vi "XY Dialog - Update Selected Paths.vi"(7 "Data":variant, 8 "error in (no error)":errorcluster, 9 "Type":T1, 10 "Tree Browser Refnun":refnum<k24>, 11 "Dialog Data in":T2={"GraphData"={"Custom Data"=variant, "EventRegs"={"SystemChange"=refnum, "WorkspaceState"=refnum, "Graph"=refnum, "Wks&Dialog&Periodic"=refnum}, "References"={"X.Scale.Auto"=refnum, "Y.Scale.Auto"=refnum, "X.Scale.Once"=refnum, "Y.Scale.Once"=refnum, "LegendVis"=refnum, "Graph"=refnum}, "Persistent Data"={"Label"="", "Graph Props"={"Plots"=[], "Legend:Number of Rows"=0, "Scale Properties"={"X.Auto"=FALSE, "X.Min"=0.0, "X.Max"=0.0, "X.IgnoreTS"=FALSE, "X.Precision"=0, "X.Label:"="", "X.LabelVis"=FALSE, "X.DefLabel"=FALSE, "Y.Auto"=FALSE, "Y.Min"=0.0, "Y.Max"=0.0, "Y.Format"=0, "Y.Precision:"=0, "Y.Label:"="", "Y.LabelVis"=FALSE, "Y.DefLabel"=FALSE, "X.Format"=0}, "Legend:Visible"=TRUE, "BgColor"=0, "Last Plot Width"=0, "Resize"=FALSE}, "UDP Data"={"Decimation"=0, "UDP Buffer Size"=0, "History Length"=0.0, "Update Rate"=enum."15 Hz", "Channel Paths"=[], "Channel Names"=[]}}, "System"={"To Workspace"=refnum, "From Workspace"=refnum, "NIVS helper"=refnum, "Gtwy"="", "Root"=refnum, "Workspace"=refnum, "SystemStateRefs"={"CustDatRef"=refnum, "EvtRef"=refnum, "Target State User Event"=refnum}, "Connected?"=FALSE, "FromDialog"=refnum, "ErrFlag"=FALSE, "New"=FALSE, "ErrState"="", "Save"=FALSE, "Hold"=FALSE, "Periodic"=refnum, "ToDialog"=refnum, "DialogEventReg"=refnum, "UseSavedWidth"=FALSE, "TreeBrowserEventReg"=refnum, "UDPChannelStreamSession"=refnum, "Valid Channels?"=FALSE, "Update Graph"=refnum, "UDP Queue"=refnum, "Graph Update Queue"=refnum}, "GraphData"=[], "UDP Stream Active?"=FALSE}, "References"={"BgColor"=refnum, "Title"=refnum, "Waveforms"=refnum, "PointsPerPixel"=refnum, "Low"=refnum, "High"=refnum, "History"=refnum, "N"=refnum, "M"=refnum, "IgnTimeStamp"=refnum, "X.Precision"=refnum, "X.Label"=refnum, "X.Label.Default"=refnum, "X.Label.Visible"=refnum, "X.Autoscale"=refnum, "X.Max"=refnum, "X.Min"=refnum, "Y.Format"=refnum, "Y.Precision"=refnum, "Y.Label"=refnum, "Y.Label.Default"=refnum, "Y.Label.Visible"=refnum, "Y.Autoscale"=refnum, "Y.Max"=refnum, "Y.Min"=refnum, "rate"=refnum, "path"=refnum, "Alias TreeBrowser"=refnum, "Y Channel Listbox"=refnum, "X Channel Listbox"=refnum, "X.Format"=refnum, "X Next"=refnum, "Y Next"=refnum, "X Previous"=refnum, "Y Previous"=refnum, "Decimation"=refnum, "History Length"=refnum, "UDP Buffer Size"=refnum}, "Tree Selected Paths"=[], "SelectedIdx"=0, "dts"=[], "X Selected Paths"=[], "Y Selected Paths"=[]} {"GraphData"."Persistent Data"."Graph Props"."Scale Properties"."X.Format" items=["Decimal", "Scientific", "Engineering", "Binary", "Octal", "Hexadecimal", "Relative Time", "Time and Date", "SI", "Automatic"]; "GraphData"."Persistent Data"."Graph Props"."Scale Properties"."Y.Precision:" items=["0", "1", "2", "3", "4", "5", "6", "7"]; "GraphData"."Persistent Data"."Graph Props"."Scale Properties"."Y.Format" items=["Decimal", "Scientific", "Engineering", "Binary", "Octal", "Hexadecimal", "Relative Time", "Time and Date", "SI", "Automatic"]; "GraphData"."Persistent Data"."Graph Props"."Scale Properties"."X.Precision" items=["0", "1", "2", "3", "4", "5", "6", "7"]}) -> (0 "error out":errorcluster, 3 "Dialog Data out":T2={"GraphData"={"Custom Data"=variant, "EventRegs"={"SystemChange"=refnum, "WorkspaceState"=refnum, "Graph"=refnum, "Wks&Dialog&Periodic"=refnum}, "References"={"X.Scale.Auto"=refnum, "Y.Scale.Auto"=refnum, "X.Scale.Once"=refnum, "Y.Scale.Once"=refnum, "LegendVis"=refnum, "Graph"=refnum}, "Persistent Data"={"Label"="", "Graph Props"={"Plots"=[], "Legend:Number of Rows"=0, "Scale Properties"={"X.Auto"=FALSE, "X.Min"=0.0, "X.Max"=0.0, "X.IgnoreTS"=FALSE, "X.Precision"=0, "X.Label:"="", "X.LabelVis"=FALSE, "X.DefLabel"=FALSE, "Y.Auto"=FALSE, "Y.Min"=0.0, "Y.Max"=0.0, "Y.Format"=0, "Y.Precision:"=0, "Y.Label:"="", "Y.LabelVis"=FALSE, "Y.DefLabel"=FALSE, "X.Format"=0}, "Legend:Visible"=TRUE, "BgColor"=0, "Last Plot Width"=0, "Resize"=FALSE}, "UDP Data"={"Decimation"=0, "UDP Buffer Size"=0, "History Length"=0.0, "Update Rate"=enum."15 Hz", "Channel Paths"=[], "Channel Names"=[]}}, "System"={"To Workspace"=refnum, "From Workspace"=refnum, "NIVS helper"=refnum, "Gtwy"="", "Root"=refnum, "Workspace"=refnum, "SystemStateRefs"={"CustDatRef"=refnum, "EvtRef"=refnum, "Target State User Event"=refnum}, "Connected?"=FALSE, "FromDialog"=refnum, "ErrFlag"=FALSE, "New"=FALSE, "ErrState"="", "Save"=FALSE, "Hold"=FALSE, "Periodic"=refnum, "ToDialog"=refnum, "DialogEventReg"=refnum, "UseSavedWidth"=FALSE, "TreeBrowserEventReg"=refnum, "UDPChannelStreamSession"=refnum, "Valid Channels?"=FALSE, "Update Graph"=refnum, "UDP Queue"=refnum, "Graph Update Queue"=refnum}, "GraphData"=[], "UDP Stream Active?"=FALSE}, "References"={"BgColor"=refnum, "Title"=refnum, "Waveforms"=refnum, "PointsPerPixel"=refnum, "Low"=refnum, "High"=refnum, "History"=refnum, "N"=refnum, "M"=refnum, "IgnTimeStamp"=refnum, "X.Precision"=refnum, "X.Label"=refnum, "X.Label.Default"=refnum, "X.Label.Visible"=refnum, "X.Autoscale"=refnum, "X.Max"=refnum, "X.Min"=refnum, "Y.Format"=refnum, "Y.Precision"=refnum, "Y.Label"=refnum, "Y.Label.Default"=refnum, "Y.Label.Visible"=refnum, "Y.Autoscale"=refnum, "Y.Max"=refnum, "Y.Min"=refnum, "rate"=refnum, "path"=refnum, "Alias TreeBrowser"=refnum, "Y Channel Listbox"=refnum, "X Channel Listbox"=refnum, "X.Format"=refnum, "X Next"=refnum, "Y Next"=refnum, "X Previous"=refnum, "Y Previous"=refnum, "Decimation"=refnum, "History Length"=refnum, "UDP Buffer Size"=refnum}, "Tree Selected Paths"=[], "SelectedIdx"=0, "dts"=[], "X Selected Paths"=[], "Y Selected Paths"=[]} {"GraphData"."Persistent Data"."Graph Props"."Scale Properties"."X.Format" items=["Decimal", "Scientific", "Engineering", "Binary", "Octal", "Hexadecimal", "Relative Time", "Time and Date", "SI", "Automatic"]; "GraphData"."Persistent Data"."Graph Props"."Scale Properties"."Y.Precision:" items=["0", "1", "2", "3", "4", "5", "6", "7"]; "GraphData"."Persistent Data"."Graph Props"."Scale Properties"."Y.Format" items=["Decimal", "Scientific", "Engineering", "Binary", "Octal", "Hexadecimal", "Relative Time", "Time and Date", "SI", "Automatic"]; "GraphData"."Persistent Data"."Graph Props"."Scale Properties"."X.Precision" items=["0", "1", "2", "3", "4", "5", "6", "7"]})   [LabVIEW 2020, in "Workspace MultiY Graph.lvlib"]
uses:
  Workspace MultiY Graph.lvlib
  XY Top level dialog data.ctl
  XY Top level workspace graph data.ctl
  <vilib>/NI VeriStand/Execution/Workspace/SystemStateRegEventRef.ctl
  <vilib>/NI VeriStand/Execution/Workspace/Target State Info.ctl
  <vilib>/NI VeriStand/Execution/Workspace/Target State.ctl
  <vilib>/NI VeriStand/Display Template Support/DisplayTemplateSupport.llb/enum_Display Template Handler Minimal To Widget Msg.ctl
  XY Dialog Msg to Control.ctl
  XY Dialog Msg Type.ctl
  XY Persistent Data.ctl
  XY Graph Properties.ctl
  XY Plot Properties.ctl
  XY Scale Properties.ctl
  XY Scale Precision.ctl
  XY Scale Format.ctl
  UDP Data.ctl
  Update Rate.ctl
  XY References.ctl
  <vilib>/NI VeriStand/Display Template Support/DisplayTemplateSupport.llb/enum_Display Template Handler Minimal To Workspace.ctl
  NationalInstruments.VeriStand.SystemStorage
  <vilib>/NI VeriStand/Execution/Workspace/WorkspaceAPI.ctl
  NationalInstruments.VeriStand.ClientAPI
  <vilib>/NI VeriStand/Execution/Workspace/SystemStateEventRef.ctl
  XY Control Msg to Dialog.ctl
  <vilib>/NI VeriStand/UI Controls/Tree and Alias Browser/Net Event Data Ref.ctl
  <vilib>/NI VeriStand/UI Controls/Tree and Alias Browser/Net Event Data.ctl
  <vilib>/NI VeriStand/UI Controls/Tree and Alias Browser/Net Event.ctl
  <vilib>/NI VeriStand/Execution/Workspace/UDPChannelStreamSession.ctl
  UDP Queue Data.ctl
  UDP Action State.ctl
  Graph Update Queue Data.ctl
  Graph Update Action State.ctl
  XY Dialog References.ctl
  NationalInstruments.VeriStand.SystemStorageUI
  <vilib>/NI VeriStand/UI Controls/Tree and Alias Browser/NI_VS UI Tree Alias Browser.lvlib
  <vilib>/NI VeriStand/Execution/Workspace/NI_VS Workspace ExecutionAPI.lvlib
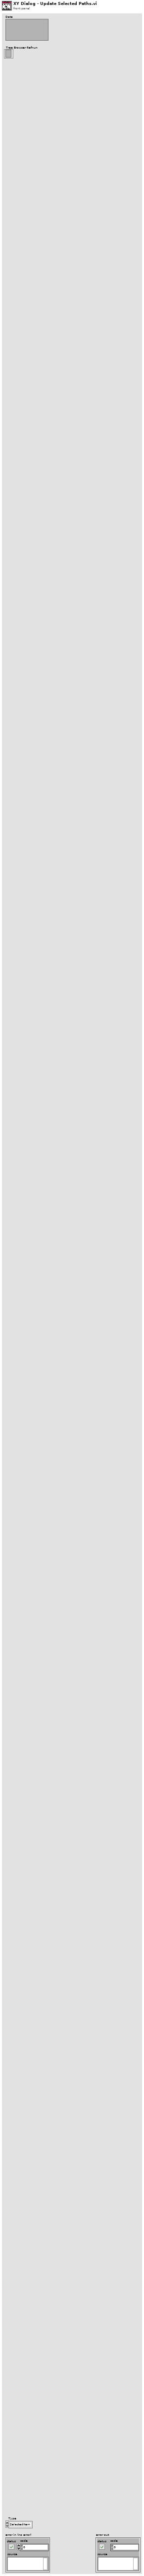
[diagram p1: front panel]
types:
  T1 = typedef "NI_VS UI Tree Alias Browser.lvlib/Net Event.ctl" = enum16{"SelectedItem", "DblClick"}
  T2 = typedef "Workspace MultiY Graph.lvlib/XY Top level dialog data.ctl" = cluster{"GraphData":T3, "References":T17, "Tree Selected Paths":string[][], "SelectedIdx":i32, "dts":dbl[], "X Selected Paths":string[][], "Y Selected Paths":string[][]}
  T3 = typedef "Workspace MultiY Graph.lvlib/XY Top level workspace graph data.ctl" = cluster{"Custom Data":variant, "EventRegs":cluster{"SystemChange":T4, "WorkspaceState":refnum<event-registration>, "Graph":refnum<event-registration>, "Wks&Dialog&Periodic":refnum<event-registration>}, "References":T5, "Persistent Data":T6, "System":cluster{"To Workspace":refnum<user-event>, "From Workspace":refnum<user-event>, "NIVS helper":refnum<vi>, "Gtwy":string, "Root":refnum<k24>, "Workspace":T14, "SystemStateRefs":T15, "Connected?":bool, "FromDialog":refnum<user-event>, "ErrFlag":bool, "New":bool, "ErrState":string, "Save":bool, "Hold":bool, "Periodic":refnum<user-event>, "ToDialog":refnum<user-event>, "DialogEventReg":refnum<event-registration>, "UseSavedWidth":bool, "TreeBrowserEventReg":refnum<event-registration>, "UDPChannelStreamSession":T16, "Valid Channels?":bool, "Update Graph":refnum<user-event>, "UDP Queue":refnum<queue>, "Graph Update Queue":refnum<queue>}, "GraphData":cluster{"X":dbl[], "Y":dbl[]}[], "UDP Stream Active?":bool}
  T4 = typedef "NI_VS Workspace ExecutionAPI.lvlib/SystemStateRegEventRef.ctl" = refnum<event-registration>
  T5 = typedef "Workspace MultiY Graph.lvlib/XY References.ctl" = cluster{"X.Scale.Auto":refnum<vi>, "Y.Scale.Auto":refnum<vi>, "X.Scale.Once":refnum<vi>, "Y.Scale.Once":refnum<vi>, "LegendVis":refnum<vi>, "Graph":refnum<vi>}
  T6 = typedef "Workspace MultiY Graph.lvlib/XY Persistent Data.ctl" = cluster{"Label":string, "Graph Props":T7, "UDP Data":T12}
  T7 = typedef "Workspace MultiY Graph.lvlib/XY Graph Properties.ctl" = cluster{"Plots":T8[], "Legend:Number of Rows":u32, "Scale Properties":T9, "Legend:Visible":bool, "BgColor":u32, "Last Plot Width":u32, "Resize":bool}
  T8 = typedef "Workspace MultiY Graph.lvlib/XY Plot Properties.ctl" = cluster{"Bar Plot Style":u8, "Digital Line Style":u8, "Digital Transition Location":u8, "Digital Transition Type":u8, "Fill To":i16, "Fill/Point Color":u32, "Label Format":u8, "Line Style":u8, "Line Width":u8, "Plot Color":u32, "Plot Interpolation":u8, "Point Style":u8, "Visible":bool, "X Scale Index":u32, "Y Scale Index":u32}
  T9 = typedef "Workspace MultiY Graph.lvlib/XY Scale Properties.ctl" = cluster{"X.Auto":bool, "X.Min":dbl, "X.Max":dbl, "X.IgnoreTS":bool, "X.Precision":T10, "X.Label:":string, "X.LabelVis":bool, "X.DefLabel":bool, "Y.Auto":bool, "Y.Min":dbl, "Y.Max":dbl, "Y.Format":T11, "Y.Precision:":T10, "Y.Label:":string, "Y.LabelVis":bool, "Y.DefLabel":bool, "X.Format":T11}
  T10 = typedef "Workspace MultiY Graph.lvlib/XY Scale Precision.ctl" = u8
  T11 = typedef "Workspace MultiY Graph.lvlib/XY Scale Format.ctl" = u8
  T12 = typedef "Workspace MultiY Graph.lvlib/UDP Data.ctl" = cluster{"Decimation":i32, "UDP Buffer Size":u32, "History Length":dbl, "Update Rate":T13, "Channel Paths":string[], "Channel Names":string[]}
  T13 = typedef "Workspace MultiY Graph.lvlib/Update Rate.ctl" = enum8{"15 Hz", "10 Hz", "5 Hz", "4 Hz", "3 Hz", "2 Hz", "1 Hz", "0.5 Hz"}
  T14 = typedef "NI_VS Workspace ExecutionAPI.lvlib/WorkspaceAPI.ctl" = refnum<k24>
  T15 = typedef "NI_VS Workspace ExecutionAPI.lvlib/SystemStateEventRef.ctl" = cluster{"CustDatRef":refnum<user-event>, "EvtRef":refnum<k27>, "Target State User Event":refnum<user-event>}
  T16 = typedef "NI_VS Workspace ExecutionAPI.lvlib/UDPChannelStreamSession.ctl" = refnum<k24>
  T17 = typedef "Workspace MultiY Graph.lvlib/XY Dialog References.ctl" = cluster{"BgColor":refnum<vi>, "Title":refnum<vi>, "Waveforms":refnum<vi>, "PointsPerPixel":refnum<vi>, "Low":refnum<vi>, "High":refnum<vi>, "History":refnum<vi>, "N":refnum<vi>, "M":refnum<vi>, "IgnTimeStamp":refnum<vi>, "X.Precision":refnum<vi>, "X.Label":refnum<vi>, "X.Label.Default":refnum<vi>, "X.Label.Visible":refnum<vi>, "X.Autoscale":refnum<vi>, "X.Max":refnum<vi>, "X.Min":refnum<vi>, "Y.Format":refnum<vi>, "Y.Precision":refnum<vi>, "Y.Label":refnum<vi>, "Y.Label.Default":refnum<vi>, "Y.Label.Visible":refnum<vi>, "Y.Autoscale":refnum<vi>, "Y.Max":refnum<vi>, "Y.Min":refnum<vi>, "rate":refnum<vi>, "path":refnum<vi>, "Alias TreeBrowser":refnum<vi>, "Y Channel Listbox":refnum<vi>, "X Channel Listbox":refnum<vi>, "X.Format":refnum<vi>, "X Next":refnum<vi>, "Y Next":refnum<vi>, "X Previous":refnum<vi>, "Y Previous":refnum<vi>, "Decimation":refnum<vi>, "History Length":refnum<vi>, "UDP Buffer Size":refnum<vi>}
  T18 = enum8{"Enabled", "Disabled", "Disabled and Grayed Out"}
  T19 = typedef "NI_VS UI Tree Alias Browser.lvlib/Node Ref.ctl" = refnum<k24>
  T20 = enum8{"Enabled", "Disabled", "Disabled and Grayed Out"}[]
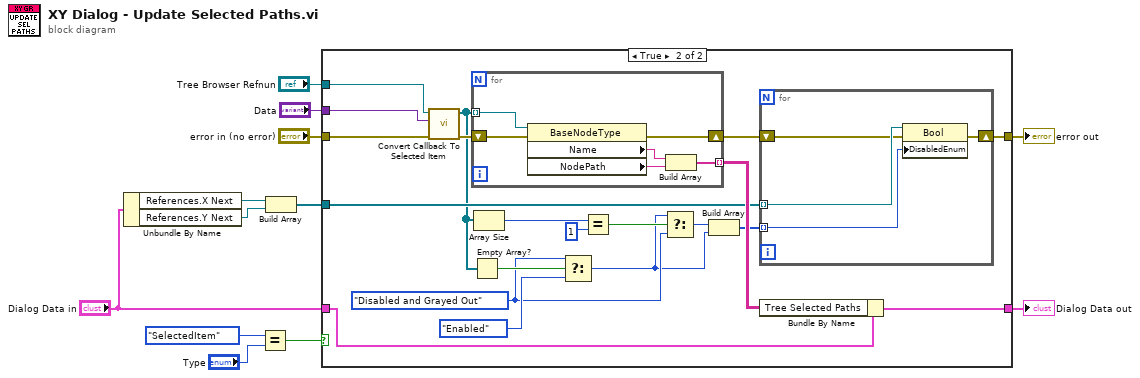
[diagram p0: block diagram]
diagram:
  n1 = Unbundle By Name("Dialog Data in") -> ("References.X Next"=w10:refnum<vi>, "References.Y Next"=w11:refnum<vi>)
  n2 = Equal?(x=Net_Event."SelectedItem", y="Type") -> (x = y?=w7:bool)
  n3 = Build Array(w10, w11) -> (w12:refnum<vi>[])
  n4 = case shown="True" w7 {
    tunnel: "Tree Browser Refnun" -> [_ w34]
    tunnel: "error in (no error)" -> [w13 w33]
    tunnel: "Data" -> [_ w32]
    tunnel: [w13 w25] -> w4
    tunnel: "Dialog Data in" -> [w14 w30]
    tunnel: [w14 w29] -> w8
    tunnel: w12 -> [_ w27]
    frame False {
    }
    frame True {
      w18 = T18."Disabled and Grayed Out" ("Disabled")
      n5 = call <vilib>:"Convert Callback To Selected Item.vi"("error in"=w33, "Data"=w32, "TreeAliasBrowser Ref"=w34) -> ("error out"=w31:errorcluster, "Selected Items"=w22:T19[])  [unwired: 7 in]
      n6 = for {
        tunnel: w22 -> [w44] mode=indexing
        shift-right: [w42] -> w26
        shift-left: w31 -> [w43]
        tunnel: [w39] -> w28 mode=indexing
        n7 = property class="BaseNodeType"(reference=w44, error in=w43) -> (error out=w42:errorcluster, "Name"=w41:string, "NodePath"=w40:string)  [unwired: 1 out]
        n8 = Build Array(w41, w40) -> (w39:string[])
      }
      n9 = Empty Array?(array=w22) -> (empty?=w24:bool)
      n10 = Array Size(array=w22) -> (size(s)=w21:i32)
      n11 = Select(t=w18, s=w24, f=T18."Enabled" ("Disabled")) -> (s? t:f=w16:T18)
      n12 = Equal?(x=w21, y=1) -> (x = y?=w19:bool)
      n13 = Select(t=w16, s=w19, f=w18) -> (s? t:f=w17:T18)
      n14 = Build Array(w17, w16) -> (w15:T20)
      n15 = for {
        tunnel: w27 -> [w38] mode=indexing
        shift-right: [w36] -> w25
        shift-left: w26 -> [w37]
        tunnel: w15 -> [w35] mode=indexing
        n16 = property class="Bool"(reference=w38, error in=w37, "DisabledEnum"=w35) -> (error out=w36:errorcluster)  [unwired: 1 out]
      }
      n17 = Bundle By Name(cluster=w30, "Tree Selected Paths"=w28) -> (w29:T2)
    }
  }
  "Dialog Data out" <- w8
  "error out" <- w4
